vi "Example Callback.vi"(8 "error in (no error)":errorcluster, 9 "Scope":variant, 11 "Value":variant) -> (0 "error out":errorcluster)   [LabVIEW 2017, in "Basic Example.lvlib"]
uses:
  Basic Example.lvlib
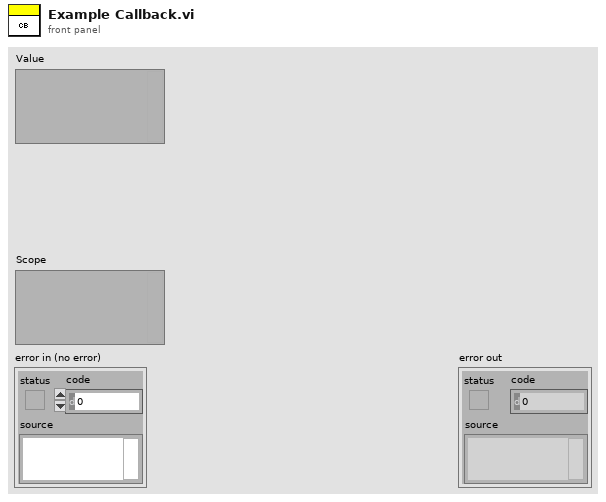
[diagram p1: front panel]
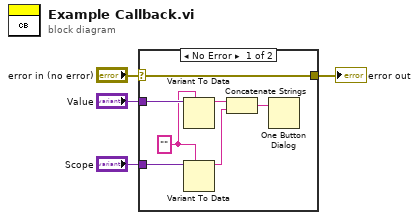
[diagram p0: block diagram]
diagram:
  n1 = case shown="No Error" "error in (no error)" {
    selector: "error in (no error)" -> [w11 w12]
    tunnel: [w11 w12] -> w3
    tunnel: "Scope" -> [w9 _]
    tunnel: "Value" -> [w10 _]
    frame No Error {
      w8 = ""
      n2 = Variant To Data(type=w8, Variant=w10) -> (data=w7:string)  [unwired: 1 in, 1 out]
      n3 = Variant To Data(type=w8, Variant=w9) -> (data=w6:string)  [unwired: 1 in, 1 out]
      n4 = Concatenate Strings(w7, w6) -> (w5:string)
      n5 = One Button Dialog(message=w5) -> ()  [unwired: 1 in, 1 out]
    }
    frame Error {
    }
  }
  "error out" <- w3
